vi "ProcessHandshakeResponse.vi"(0 "HTTP Headers":string, 7 "Sec-WebSocket-Key":string, 11 "error in (no error)":errorcluster) -> (4 "Is Websocket Response?":bool, 8 "Response Status Code":T1=101 items=["Switching Protocols"=101, "Bad Request"=400, "Forbidden"=403, "Not Found"=404, "Upgrade Required"=426], 14 "Headers Out":variant, 15 "error out":errorcluster)   [LabVIEW 2021, in "LV WebSockets.lvlib"]
doc: "Processes the server handshake response. Converts the raw HTTP header string into it's main component parts needed to check if the server response is a valid websocket handshake response. The additional headers are returned in a variant lookup table."
uses:
  LV WebSockets.lvlib
  HTTPResponseCodes.ctl
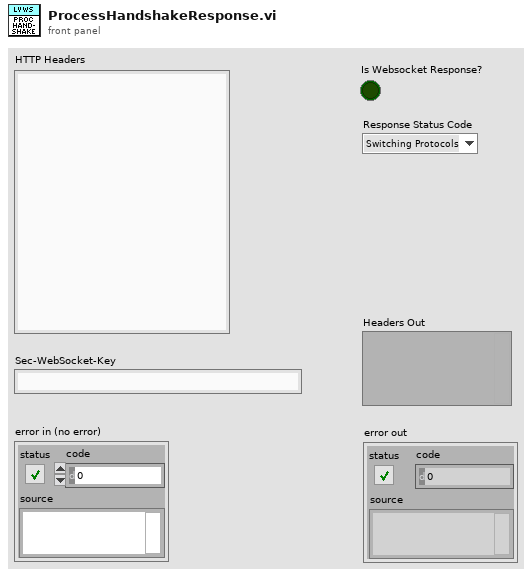
[diagram p1: front panel]
types:
  T1 = typedef "LV WebSockets.lvlib/HTTPResponseCodes.ctl" = u16
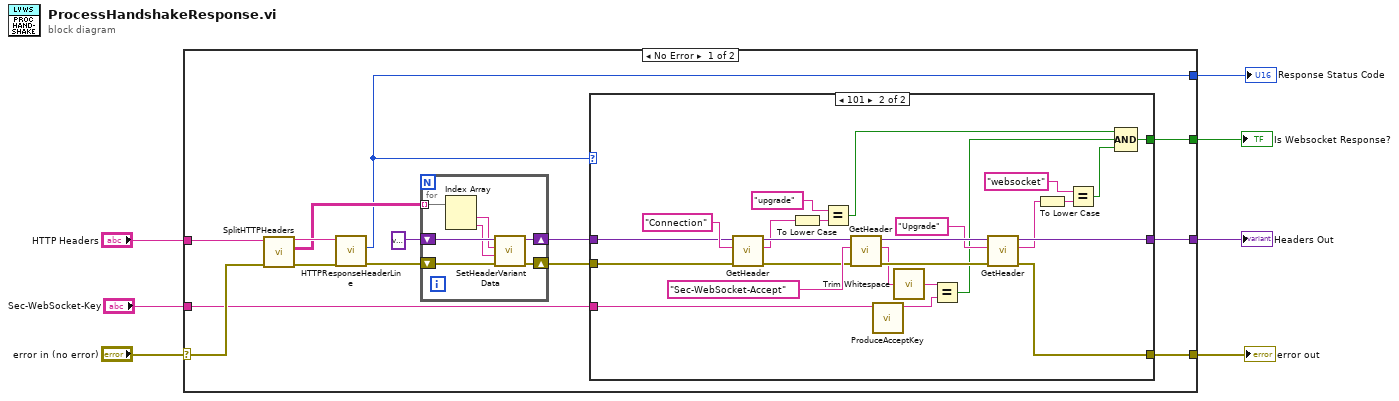
[diagram p0: block diagram]
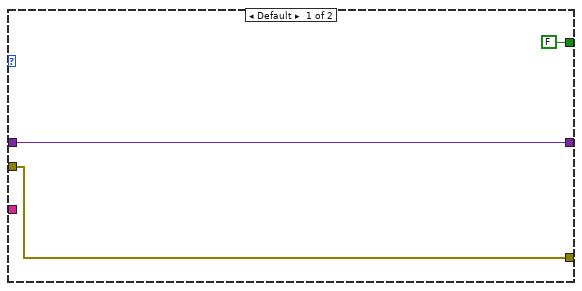
[diagram p2: hidden frame]
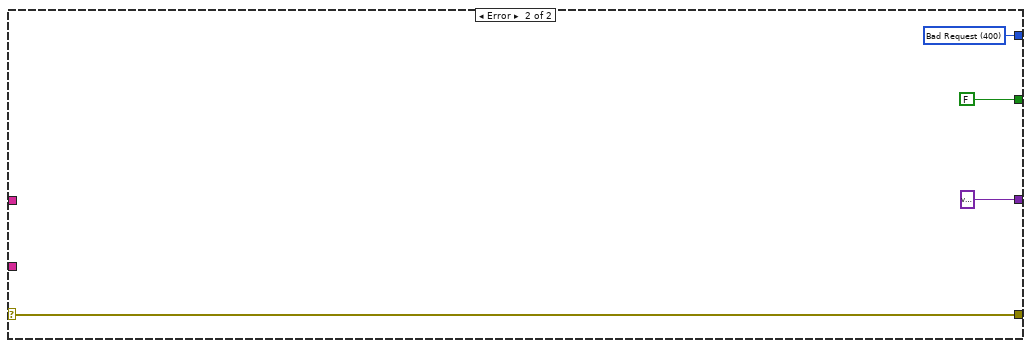
[diagram p3: hidden frame]
diagram:
  n1 = case shown="No Error" "error in (no error)" {
    selector: "error in (no error)" -> [w18 w60]
    tunnel: "HTTP Headers" -> [w21 _]
    tunnel: [w20 variant ("Headers Out")] -> w6
    tunnel: [w19 FALSE] -> w5
    tunnel: [w17 w60] -> w3
    tunnel: "Sec-WebSocket-Key" -> [w14 _]
    tunnel: [w8 w57] -> w1
    frame No Error {
      n2 = call "SplitHTTPHeaders.vi"("error in (no error)"=w18, "HTTP Header String"=w21) -> ("error out"=w16:errorcluster, "Headers Array"=w9:string[][], "HTTP Request"=w15:string)  [unwired: 7 in]
      n3 = call "HTTPResponseHeaderLine.vi"("error in (no error)"=w16, "HTTP Request Line"=w15) -> ("error out"=w13:errorcluster, "Status Code"=w8:T1)  [unwired: 6 in, 2 out]
      n4 = for {
        tunnel: w9 -> [w28] mode=indexing
        shift-right: [w27] -> w10
        shift-left: variant -> [w24]
        shift-right: [w26] -> w12
        shift-left: w13 -> [w25]
        n5 = Index Array(array=w28) -> (element #1=w23:string, element #2=w22:string)  [unwired: 2 in]
        n6 = call "SetHeaderVariantData.vi"("error in (no error)"=w25, "Value"=w22, "Name"=w23, "Variant in"=w24) -> ("error out"=w26:errorcluster, "Variant out"=w27:variant)  [unwired: 6 in]
      }
      n7 = case shown="101" w8 {
        tunnel: [w30 w52] -> w20
        tunnel: [FALSE w48] -> w19
        tunnel: [w29 w45] -> w17
        tunnel: w12 -> [w29 w34]
        tunnel: w14 -> [_ w38]
        tunnel: w10 -> [w30 w35]
        frame Default {
        }
        frame 101 {
          n8 = call "GetHeader.vi"("error in (no error)"=w34, "Name"="Connection" ("name"), "Headers In"=w35) -> ("error out"=w47:errorcluster, "Data"=w40:string, "Headers Out"=w55:variant)  [unwired: 5 in, 1 out]
          n9 = To Lower Case(string=w40) -> (all lower case string=w41:string)
          n10 = Equal?(x="upgrade", y=w41) -> (x = y?=w39:bool)
          n11 = call "GetHeader.vi"("error in (no error)"=w47, "Name"="Sec-WebSocket-Accept", "Headers In"=w55) -> ("error out"=w46:errorcluster, "Data"=w32:string, "Headers Out"=w53:variant)  [unwired: 5 in, 1 out]
          n12 = call "ProduceAcceptKey.vi"("Sec-WebSocket-Key"=w38) -> ("Sec-WebSocket-Accept"=w37:string)  [unwired: 10 in]
          n13 = call <vilib>:"Trim Whitespace.vi"("string"=w32) -> ("trimmed string"=w33:string)  [unwired: 1 in]
          n14 = Equal?(x=w33, y=w37) -> (x = y?=w36:bool)
          n15 = call "GetHeader.vi"("error in (no error)"=w46, "Name"="Upgrade", "Headers In"=w53) -> ("error out"=w45:errorcluster, "Data"=w44:string, "Headers Out"=w52:variant)  [unwired: 5 in, 1 out]
          n16 = To Lower Case(string=w44) -> (all lower case string=w43:string)
          n17 = Equal?(x="websocket", y=w43) -> (x = y?=w49:bool)
          n18 = Compound Arithmetic op=AND(w39, w36, w49) -> (w48:bool)
        }
      }
    }
    frame Error {
      w57 = T1 400 items=["Switching Protocols"=101, "Bad Request"=400, "Forbidden"=403, "Not Found"=404, "Upgrade Required"=426] ("Status Code")
    }
  }
  "Is Websocket Response?" <- w5
  "Headers Out" <- w6
  "error out" <- w3
  "Response Status Code" <- w1
